vi "Initialize (Core).vi"(0 "resources":string, 1 "https?":bool, 2 "slsc type":T1, 5 "Hostname/IP":string, 7 "Port":u16, 11 "error in (no error)":errorcluster, 12 "username":string, 13 "password":string) -> (4 "SLSC Remote out":refnum<class "SLSC Remote.lvclass">, 15 "error out":errorcluster)   [LabVIEW 2015, in "SLSC Remote.lvclass"]
uses:
  SLSC Remote.lvclass
  SLSC Interface Class/slsc type.ctl
  <vilib>/httpClient/POSTBuffer.vi
  <vilib>/NI/i3 JSON/JSON Parsing/Get Object Parameter Files/Get Object Parameter - String.vi
  <vilib>/httpClient/LabVIEWHTTPClient.lvlib
  <vilib>/NI/i3 JSON/i3-json.lvlib
  <vilib>/NI/NI JSONRPC Server Framework/Classes/Server/JSONRPC Server.lvclass
  SLSC Interface Class/SLSC Interface.lvclass
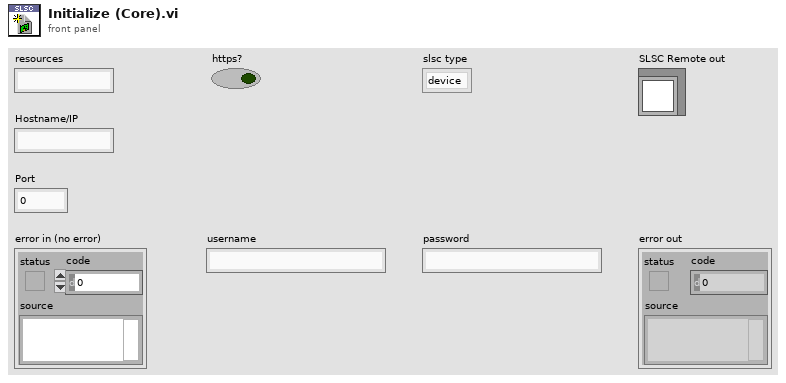
[diagram p1: front panel]
types:
  T1 = typedef "SLSC Interface.lvclass/slsc type.ctl" = enum16{"device", "nvmem", "channel", "none"}
  T2 = typedef "LabVIEWHTTPClient.lvlib/ClientHandle.ctl" = refnum<k1>
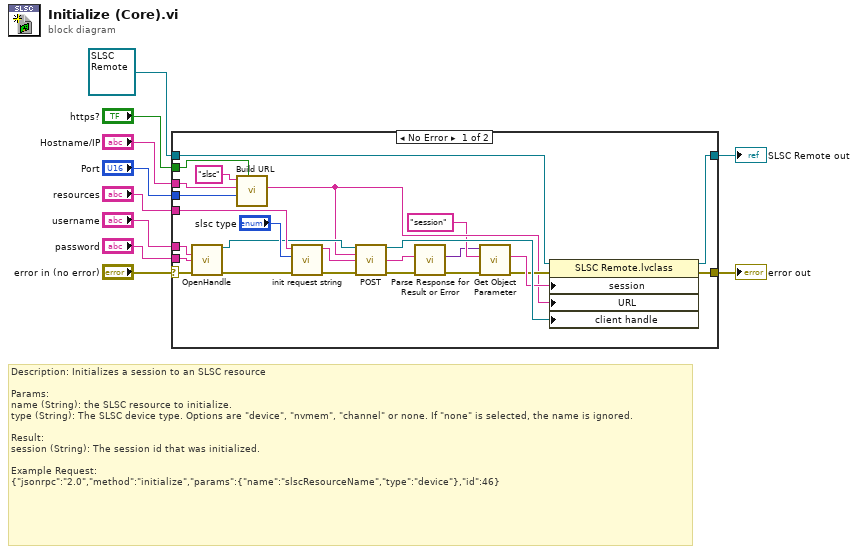
[diagram p0: block diagram]
diagram:
  # "Description: Initializes a session to an SLSC resource\n\nParams:\nname (String): the SLSC resource to initialize.\ntype (String): The SLSC device type. Options are \"device\", \"nvmem\", \"channel\" or none. If \"none\" is selected, the name is ignored.\n\nResult:\nsession (String): The session id that was initialized.\n\nExample Request: \n{\"jsonrpc\":\"2.0\",\"method\":\"initialize\",\"params\":{\"name\":\"slscResourceName\",\"type\":\"device\"},\"id\":46}"
  n1 = case shown="No Error" "error in (no error)" {
    selector: "error in (no error)" -> [w30 w37]
    tunnel: [w33 w37] -> w10
    tunnel: [w34 w36] -> w8
    tunnel: refnum<class "SLSC Remote.lvclass"> refnum ("SLSC Local in") -> [w35 w36]
    tunnel: "resources" -> [w28 _]
    tunnel: "username" -> [w32 _]
    tunnel: "password" -> [w31 _]
    tunnel: "https?" -> [w21 _]
    tunnel: "Hostname/IP" -> [w20 _]
    tunnel: "Port" -> [w19 _]
    frame No Error {
      n2 = call <vilib>:"OpenHandle.vi"("username"=w32, "password"=w31, "error in (no error)"=w30) -> ("client handle out"=w26:T2, "error out"=w25:errorcluster)  [unwired: 11 in]
      n3 = call "Build URL.vi"("https?"=w21, "Port"=w19, "Hostname/IP"=w20, "service name"="slsc") -> ("URL"=w17:string)  [unwired: 7 in]
      n4 = call "init request string.vi"("error in (no error)"=w25, "slsc type"="slsc type", "resource"=w28) -> ("error out"=w27:errorcluster, "Request String"=w18:string)  [unwired: 7 in]
      n5 = call-poly <vilib>:"POST.vi"("client handle"=w26, "url"=w17, "buffer"=w18, "error in (no error)"=w27) -> ("client handle out"=w24:T2, "body"=w16:string, "error out"=w12:errorcluster)  [unwired: 8 in, 1 out]
      n6 = call <vilib>:"Parse Response for Result or Error.vi"("error in"=w12, "Response String In"=w16) -> ("error out"=w13:errorcluster, "Result or Error Data"=w14:variant)  [unwired: 7 in, 1 out]
      n7 = call-poly <vilib>:"Get Object Parameter.vi"("error in (no error)"=w13, "Parameter Name"="session", "JSON Tree In (JSON Object)"=w14) -> ("error out"=w22:errorcluster, "String Value"=w23:string)  [unwired: 5 in, 2 out]
      n8 = property class="SLSC Remote.lvclass"(reference=w35, error in=w22, "session"=w23, "URL"=w17, "client handle"=w24) -> (reference out=w34:refnum<class "SLSC Remote.lvclass">, error out=w33:errorcluster)
    }
    frame Error {
    }
  }
  "error out" <- w10
  "SLSC Remote out" <- w8
